vi "ProdaNG.ProcessSteps.Get.vi"(8 "error in (no error)":errorcluster, 10 "processId":i32, 11 "dbHandleIn":i32) -> (0 "error out":errorcluster, 2 "ProcSteps":T1[](array[typedef]), 3 "dbHandle":i32)   [LabVIEW 2016]
doc: "This function returns a product structure for a product, which is identified by a part and a serial number.\nImportant information: The field 'individual' was taken over from the field 'allgemein' of the legacy data directly. Because of this most products have the value 0 further on and only a few the value 1. \nParameter:\nhandle is an Integer, which is returned by the function Login() at the creation of a new connection.\nwabcoPartId is the Id of the part.\nserialNumber is the serial number of the product for the part above.\nproduct is a pointer on a product structure, which is filled if the returncode is 0. The structure must be defined in the calling program.\n\nReturncodes:\n0 No error\n< 0 ORACLE Error code\n6 (ERROR_INVALID_HANDLE) in case of an invalid handle\n1403 Record does not exist"
uses:
  Controls/ProdaNG.ProcessStep.ctl
  Controls/ProdaNG.ProcessStepSize.ctl
  <vilib>/Utility/importsl/GetValueByPointer/datatype.ctl
  <vilib>/Utility/importsl/GetValueByPointer/GetValueByPointer.xnode
  prodllNG.dll
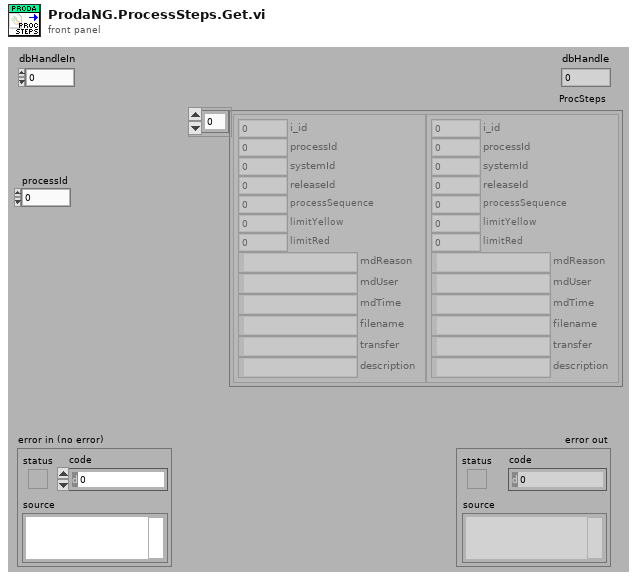
[diagram p1: front panel]
types:
  T1 = typedef "ProdaNG.ProcessStep.ctl" = cluster{"i_id":i32, "processId":i32, "systemId":i32, "releaseId":i32, "processSequence":i32, "limitYellow":dbl, "limitRed":dbl, "mdReason":string, "mdUser":string, "mdTime":string, "filename":string, "transfer":string, "description":string}
  T2 = typedef "ProdaNG.ProcessStepSize.ctl" = cluster{"i_id":i32, "processId":i32, "systemId":i32, "releaseId":i32, "processSequence":i32, "limitYellow":i32, "limitRed":i32, "mdReason":i32, "mdUser":i32, "mdTime":i32, "filename":i32, "transfer":i32, "description":i32}
  T3 = cluster{"32bit integer":i32, "LV string":string, "ProcessStep":T1}
  T4 = cluster{"32bit integer":i32, "LV string":string, "ProcessStep":T1}[]
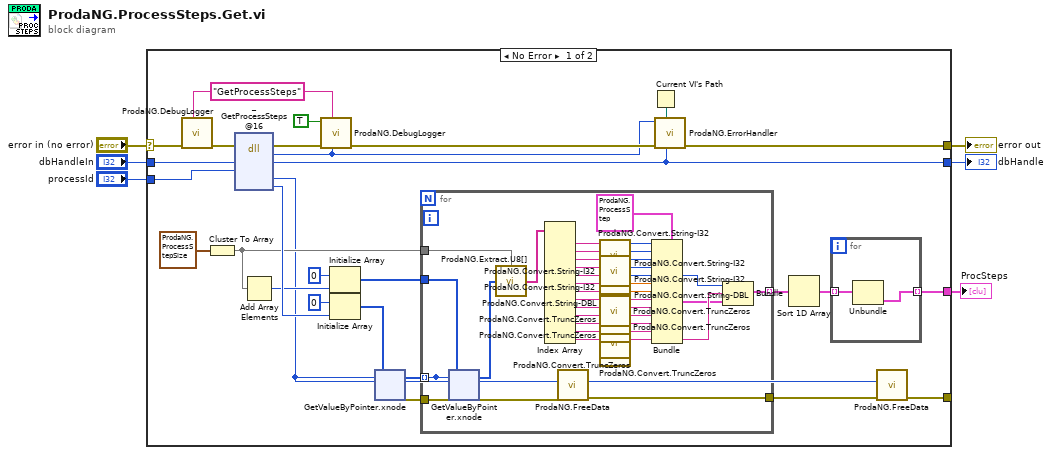
[diagram p0: block diagram]
diagram:
  n1 = case shown="No Error" "error in (no error)" {
    selector: "error in (no error)" -> [w29 w105]
    tunnel: [w34 w105] -> w5
    tunnel: "dbHandleIn" -> [w31 w104]
    tunnel: [w32 w104] -> w3
    tunnel: "processId" -> [w16 _]
    tunnel: [w7 _] -> w1
    tunnel: [w10 _] -> _
    frame No Error {
      w25 = "GetProcessSteps" ("cmd")
      n2 = call "ProdaNG.DebugLogger.vi"("cmd"=w25, "error in (no error)"=w29) -> ("error out"=w28:errorcluster)  [unwired: 9 in]
      n3 = Cluster To Array(cluster=T2 {"i_id"=4, "processId"=4, "systemId"=4, "releaseId"=4, "processSequence"=4, "limitYellow"=8, "limitRed"=8, "mdReason"=514, "mdUser"=22, "mdTime"=24, "filename"=258, "transfer"=2, "description"=514} ("ProcStepSize")) -> (array=w14:i32[])
      n4 = dll-call lib="D:/Maszup/WABCO/SVN/LineTraceSystem/SOFTWARE/sources/Database/ProdaNG/prodllNG.dll" fn="_GetProcessSteps@16" ("ProDLL wrapper.dll:ProDLL_wrapper_GetWabcoParts_GetData")(error in=w28, "dbHandle"=w31, "processId"=w16) -> (error out=w27:errorcluster, "return type"=w24:i32, "dbHandle"=w32:i32, "processSteps"=w9:u32, "countPtr"=w19:i32)  [unwired: 5 in, 1 out]
      n5 = Add Array Elements(numeric array=w14) -> (sum=w15:i32)
      n6 = call "ProdaNG.DebugLogger.vi"("return type"=w24, "cmd"=w25, "error in (no error)"=w27, "done? (F)"=TRUE) -> ("error out"=w26:errorcluster)  [unwired: 7 in]
      n7 = Initialize Array(u8 0 ("element"), w15) -> (w17:u8[])
      n8 = Initialize Array(u32 0 ("element"), w19) -> (w23:u32[])
      n9 = xnode "GetValueByPointer.xnode"("Pointer"=w9, "InputType"=w23) -> ("Output"=w20:u32[], "ErrorOut"=w21:errorcluster)  [unwired: 2 in]
      n10 = for {
        tunnel: w21 -> [w73]
        tunnel: w20 -> [w42] mode=indexing
        tunnel: w17 -> [w72]
        tunnel: w14 -> [w57]
        tunnel: [w37] -> w13 mode=indexing
        tunnel: [w41] -> w11
        n11 = xnode "GetValueByPointer.xnode"("Pointer"=w42, "InputType"=w72, "ErrorIn"=w73) -> ("Output"=w59:u8[], "ErrorOut"=w43:errorcluster)  [unwired: 1 in]
        n12 = call "ProdaNG.Extract.U8[].vi"("unsigned byte array"=w59, "Sizes"=w57) -> ("Elements"=w58:string[])
        n13 = Index Array(array=w58) -> (element #1=w61:string, element #2=w60:string, element #3=w70:string, element #4=w67:string, element #5=w64:string, element #6=w66:string, element #7=w56:string, element #8=w55:string, element #9=w52:string, element #10=w50:string, element #11=w48:string, element #12=w46:string, element #13=w44:string)  [unwired: 13 in]
        n14 = call "ProdaNG.FreeData.vi"("error in (no error)"=w43, "Pointers"=w42) -> ("error out"=w41:errorcluster)  [unwired: 9 in]
        n15 = call "ProdaNG.Convert.String-I32.vi"("unsigned byte string"=w61) -> ("32bit integer"=w63:i32)  [unwired: 10 in]
        n16 = call "ProdaNG.Convert.String-I32.vi"("unsigned byte string"=w60) -> ("32bit integer"=w62:i32)  [unwired: 10 in]
        n17 = call "ProdaNG.Convert.String-I32.vi"("unsigned byte string"=w70) -> ("32bit integer"=w69:i32)  [unwired: 10 in]
        n18 = call "ProdaNG.Convert.String-I32.vi"("unsigned byte string"=w67) -> ("32bit integer"=w68:i32)  [unwired: 10 in]
        n19 = call "ProdaNG.Convert.String-I32.vi"("unsigned byte string"=w64) -> ("32bit integer"=w39:i32)  [unwired: 10 in]
        n20 = call "ProdaNG.Convert.String-DBL.vi"("unsigned byte string"=w66) -> ("dbl integer"=w65:dbl)  [unwired: 10 in]
        n21 = call "ProdaNG.Convert.String-DBL.vi"("unsigned byte string"=w56) -> ("dbl integer"=w54:dbl)  [unwired: 10 in]
        n22 = call "ProdaNG.Convert.TruncZeros.vi"("string with \\0s"=w55) -> ("LV string"=w53:string)  [unwired: 10 in]
        n23 = call "ProdaNG.Convert.TruncZeros.vi"("string with \\0s"=w52) -> ("LV string"=w51:string)  [unwired: 10 in]
        n24 = call "ProdaNG.Convert.TruncZeros.vi"("string with \\0s"=w50) -> ("LV string"=w49:string)  [unwired: 10 in]
        n25 = call "ProdaNG.Convert.TruncZeros.vi"("string with \\0s"=w48) -> ("LV string"=w47:string)  [unwired: 10 in]
        n26 = call "ProdaNG.Convert.TruncZeros.vi"("string with \\0s"=w46) -> ("LV string"=w45:string)  [unwired: 10 in]
        n27 = call "ProdaNG.Convert.TruncZeros.vi"("string with \\0s"=w44) -> ("LV string"=w40:string)  [unwired: 10 in]
        n28 = Bundle(cluster=T1 {"i_id"=0, "processId"=0, "systemId"=0, "releaseId"=0, "processSequence"=0, "limitYellow"=0.0, "limitRed"=0.0, "mdReason"="", "mdUser"="", "mdTime"="", "filename"="", "transfer"="", "description"=""} ("ProcessStep"), "i_id"=w63, "processId"=w62, "systemId"=w69, "releaseId"=w68, "processSequence"=w39, "limitYellow"=w65, "limitRed"=w54, "mdReason"=w53, "mdUser"=w51, "mdTime"=w49, "filename"=w47, "transfer"=w45, "description"=w40) -> (w38:T1)
        n29 = Bundle("32bit integer"=w39, "LV string"=w40, "ProcessStep"=w38) -> (w37:T3)  [unwired: 1 in]
      }
      n30 = Current VI's Path() -> (path=w33:path)
      n31 = call "ProdaNG.ErrorHandler.vi"("dbHandleIn"=w32, "Path"=w33, "error in"=w26, "output_parameter"=w24) -> ("error out"=w34:errorcluster)  [unwired: 7 in]
      n32 = Sort 1D Array(array=w13) -> (sorted array=w8:T4)
      n33 = for {
        tunnel: w8 -> [w36] mode=indexing
        tunnel: [w35] -> w7 mode=indexing
        n34 = Unbundle(w36) -> ("ProcessStep"=w35:T1)  [unwired: 2 out]
      }
      n35 = call "ProdaNG.FreeData.vi"("error in (no error)"=w11, "Pointers"=w9) -> ("error out"=w10:errorcluster)  [unwired: 9 in]
    }
    frame Error {
    }
  }
  "error out" <- w5
  "dbHandle" <- w3
  "ProcSteps" <- w1
